vi "GetTime.vi"(1 "error in":errorcluster) -> (0 "Time":u32)   [LabVIEW 2015]
doc: "Gets the value from the millisecond timer. Meant to be synced with an error cluster for benchmarking."
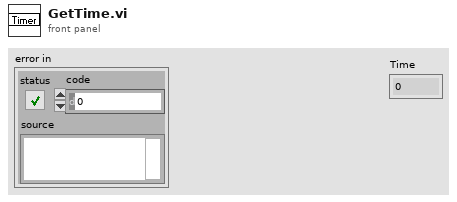
[diagram p1: front panel]
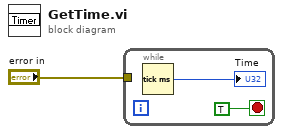
[diagram p0: block diagram]
diagram:
  n1 = while {
    tunnel: "error in" -> [_]
    stop <- TRUE stop-if-true
    n2 = Tick Count (ms)() -> (millisecond timer value=→"Time":u32)
  }
